vi "FGV Stoerungen.vi"(6 "Aktionen":T1, 9 "65-128":u64, 10 "1-64":u64, 11 "Störung aktiv?":bool[](array[boolean])) -> (1 "65-128":u64, 2 "1-64":u64, 3 "Störung aktiv?":bool[](array[boolean]))   [LabVIEW 2020, in "Stoermeldungen.lvlib"]
uses:
  Stoermeldungen.lvlib
  FGV Stoerungen Aktionen.ctl
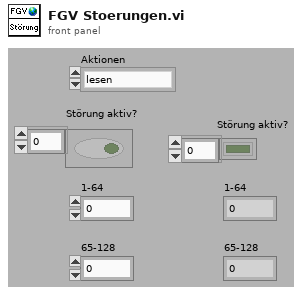
[diagram p1: front panel]
types:
  T1 = typedef "Stoermeldungen.lvlib/FGV Stoerungen Aktionen.ctl" = enum16{"lesen", "Störung aktiv?", "1-64", "65-128"}
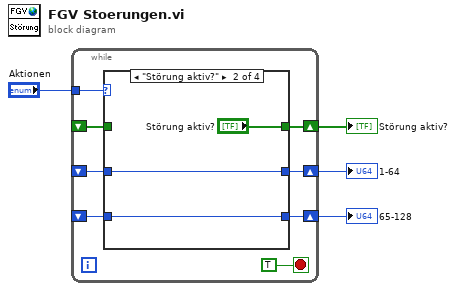
[diagram p0: block diagram]
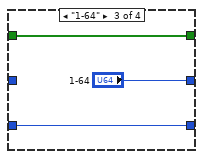
[diagram p3: hidden frame]
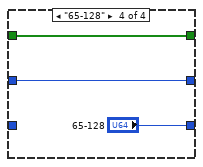
[diagram p4: hidden frame]
diagram:
  n1 = while {
    tunnel: "Aktionen" -> [w11]
    shift-right: [w5] -> w1
    shift-left: _ -> [w10]
    shift-right: [w6] -> w2
    shift-left: _ -> [w9]
    shift-right: [w7] -> w3
    shift-left: _ -> [w8]
    stop <- TRUE stop-if-true
    n2 = case shown="\"Störung aktiv?\"" w11 {
      tunnel: w10 -> [w15 _ w21 w24]
      tunnel: w9 -> [w14 w17 _ w23]
      tunnel: w8 -> [w13 w18 w20 _]
      tunnel: [w13 w18 w20 "65-128"] -> w7
      tunnel: [w14 w17 "1-64" w23] -> w6
      tunnel: [w15 "Störung aktiv?" w21 w24] -> w5
      frame "lesen", Default {
      }
      frame "Störung aktiv?" {
      }
      frame "1-64" {
      }
      frame "65-128" {
      }
    }
  }
  "1-64" <- w2
  "65-128" <- w3
  "Störung aktiv?" <- w1
